vi "UserSliderCursor (SubVI).vi"(4 "Pixel to Micron":dbl, 6 "Axes colour":u32(colorbox)=16711680, 7 "Coordinates Unit":u16(ring) items=["MM"=1, "Pixel"=0], 8 "error in (no error)":errorcluster, 9 "Image RefNum In":T1, 10 "Y slider refnum":refnum<vi>, 11 "X slider refnum":refnum<vi>) -> (0 "error out":errorcluster, 2 "Image Refnum out":T1, 3 "Cross Point":cluster{"X coordinate":dbl, "Y coordinate":dbl})   [LabVIEW 2016]
uses:
  <vilib>/vision/Image Controls.llb/IMAQ Image.ctl
panel:
  # "This subVI takes input from a pair of \nsliders to display axes on an image. \nThe Cross Point provides the \n(x,y) coordinates of the intersection\nof the two axes (in pixel units)"
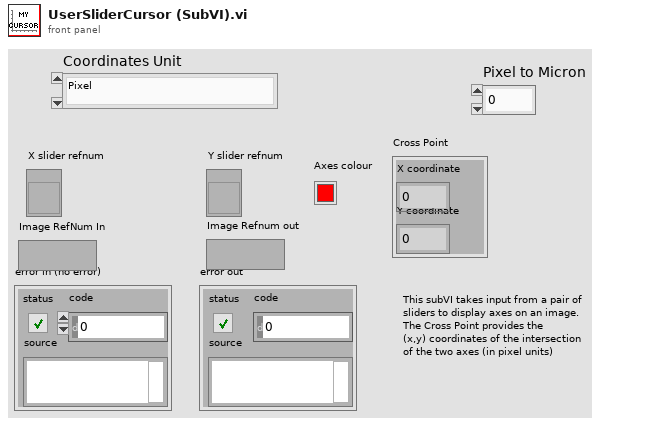
[diagram p1: front panel]
types:
  T1 = typedef "IMAQ Image.ctl" = refnum<image>
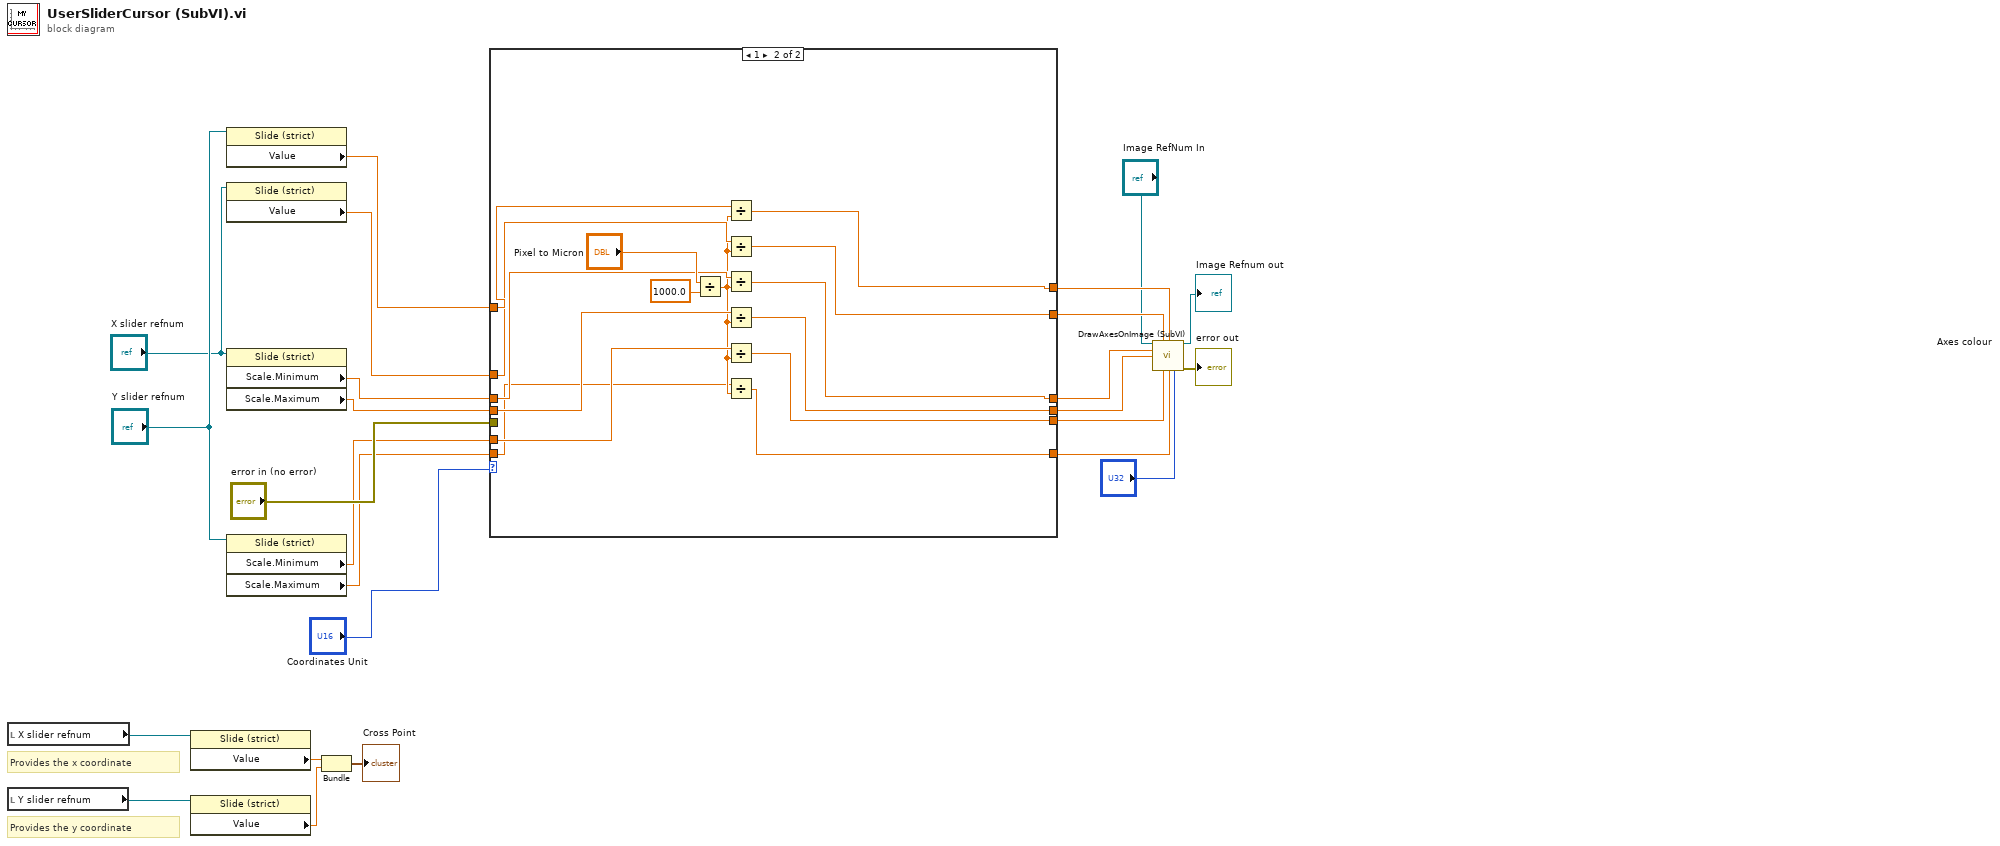
[diagram p0: block diagram]
diagram:
  # "Provides the x coordinate"
  # "Provides the y coordinate"
  n1 = local read "X slider refnum"() -> (w23:refnum<vi>)
  n2 = local read "Y slider refnum"() -> (w22:refnum<vi>)
  n3 = property class="Slide (strict)"(reference=w23) -> ("Value"=w20:dbl)  [unwired: 1 in, 2 out]
  n4 = property class="Slide (strict)"(reference=w22) -> ("Value"=w19:dbl)  [unwired: 1 in, 2 out]
  n5 = property class="Slide (strict)"(reference="Y slider refnum") -> ("Value"=w12:dbl)  [unwired: 1 in, 2 out]
  n6 = property class="Slide (strict)"(reference="X slider refnum") -> ("Value"=w13:dbl)  [unwired: 1 in, 2 out]
  n7 = property on="Property Node" class="Slide (strict)"(reference="X slider refnum") -> ("Scale.Minimum"=w14:dbl, "Scale.Maximum"=w15:dbl)  [unwired: 1 in, 2 out]
  n8 = property on="Property Node" class="Slide (strict)"(reference="Y slider refnum") -> ("Scale.Minimum"=w16:dbl, "Scale.Maximum"=w17:dbl)  [unwired: 1 in, 2 out]
  n9 = Bundle("Value"=w20, "Value"=w19) -> (→"Cross Point":cluster{"Value":dbl, "Value":dbl})  [unwired: 1 in]
  n10 = case shown="1" "Coordinates Unit" {
    tunnel: "error in (no error)" -> [_ _]
    tunnel: w17 -> [w26 w38]
    tunnel: w16 -> [w27 w40]
    tunnel: w15 -> [w28 w41]
    tunnel: w14 -> [w29 w42]
    tunnel: w13 -> [w30 w43]
    tunnel: w12 -> [w31 w44]
    tunnel: [w31 w32] -> w9
    tunnel: [w30 w33] -> w8
    tunnel: [w29 w34] -> w7
    tunnel: [w28 w35] -> w6
    tunnel: [w27 w36] -> w5
    tunnel: [w26 w37] -> w4
    frame 0, Default {
    }
    frame 1 {
      n11 = Divide(x="Pixel to Micron", y=1000.0) -> (x/y=w39:dbl)
      n12 = Divide(x=w44, y=w39) -> (x/y=w32:dbl)
      n13 = Divide(x=w43, y=w39) -> (x/y=w33:dbl)
      n14 = Divide(x=w42, y=w39) -> (x/y=w34:dbl)
      n15 = Divide(x=w41, y=w39) -> (x/y=w35:dbl)
      n16 = Divide(x=w40, y=w39) -> (x/y=w36:dbl)
      n17 = Divide(x=w38, y=w39) -> (x/y=w37:dbl)
    }
  }
  n18 = call "DrawAxesOnImage (SubVI).vi"("Image Refnum in"="Image RefNum In", "X Value"=w8, "Y Value"=w9, "X Minimum"=w7, "X Maximum"=w6, "Y Minimum"=w5, "Y Maximum"=w4, "Axes colour"="Axes colour") -> ("Image Refnum out"=→"Image Refnum out":T1, "error out"=→"error out":errorcluster)  [unwired: 6 in]
